vi "Get Configuration File Path.vi"(8 "error in (no error)":errorcluster, 11 "Configuration File Name":string) -> (0 "error out":errorcluster, 3 "Configuration File Path":path)   [LabVIEW 2024]
doc: "Gets the configuration file path in the application folder recursively."
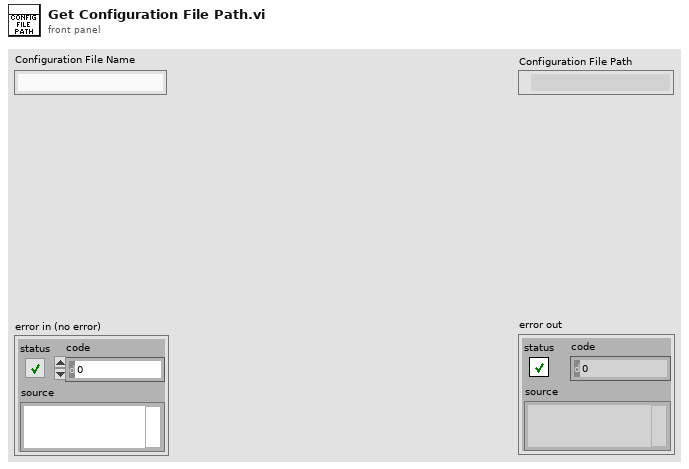
[diagram p1: front panel]
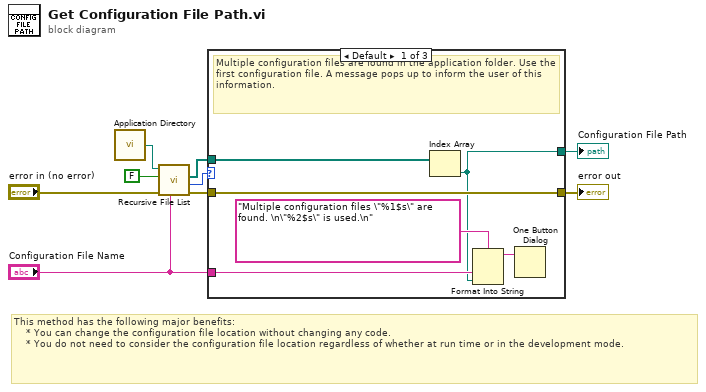
[diagram p0: block diagram]
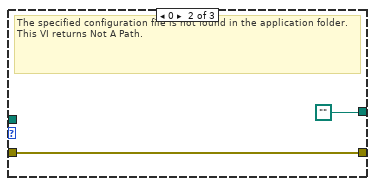
[diagram p2: hidden frame]
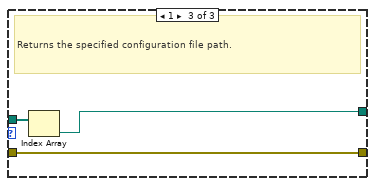
[diagram p3: hidden frame]
diagram:
  # "This method has the following major benefits:\n    * You can change the configuration file location without changing any code. \n    * You do not need to consider the configuration file location regardless of whether at run time or in the development mode."
  n1 = call <vilib>:"Application Directory.vi"() -> ("Application Directory"=w4:path)
  n2 = call <vilib>:"Recursive File List.vi"("pattern"="Configuration File Name", "error in (no error)"="error in (no error)", "Treat LLBs as Folders?"=FALSE, "Folder Path"=w4) -> ("error out"=w6:errorcluster, "Number of Files"=w7:i32, "All Files in Dir"=w1:path[])  [unwired: 3 in, 2 out]
  n3 = case shown="Default" w7 {
    tunnel: w6 -> [w15 w17 w20]
    tunnel: [w15 w17 w20] -> w5
    tunnel: "Configuration File Name" -> [w13 _ _]
    tunnel: [w11 path "" w18] -> w2
    tunnel: w1 -> [w14 _ w19]
    frame Default {
      # "Multiple configuration files are found in the application folder. Use the first configuration file. A message pops up to inform the user of this information."
      n4 = Index Array(array=w14) -> (element=w11:path)  [unwired: 1 in]
      n5 = Format Into String(format string="Multiple configuration files \"%1$s\" are found. \n\"%2$s\" is used.\n", w13, w11) -> (resulting string=w10:string)  [unwired: 2 in, 1 out]
      n6 = One Button Dialog(message=w10) -> ()  [unwired: 1 in, 1 out]
    }
    frame 0 {
      # "The specified configuration file is not found in the application folder. This VI returns Not A Path."
    }
    frame 1 {
      # "Returns the specified configuration file path."
      n7 = Index Array(array=w19) -> (element=w18:path)  [unwired: 1 in]
    }
  }
  "error out" <- w5
  "Configuration File Path" <- w2
